vi "SnapCounter_DetectEvent.vi"(3 "status":bool, 4 "error in (no error)":errorcluster, 5 "Task ID":u32) -> (0 "snap counter data":cluster{"event source":i32, "event data":u8[]}, 1 "error out":errorcluster, 2 "Task ID out":u32)   [LabVIEW 2015]
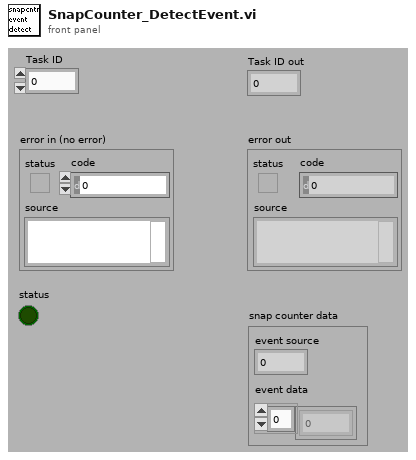
[diagram p1: front panel]
types:
  T1 = cluster{"snap event source":i32, "snap data":i32[]}
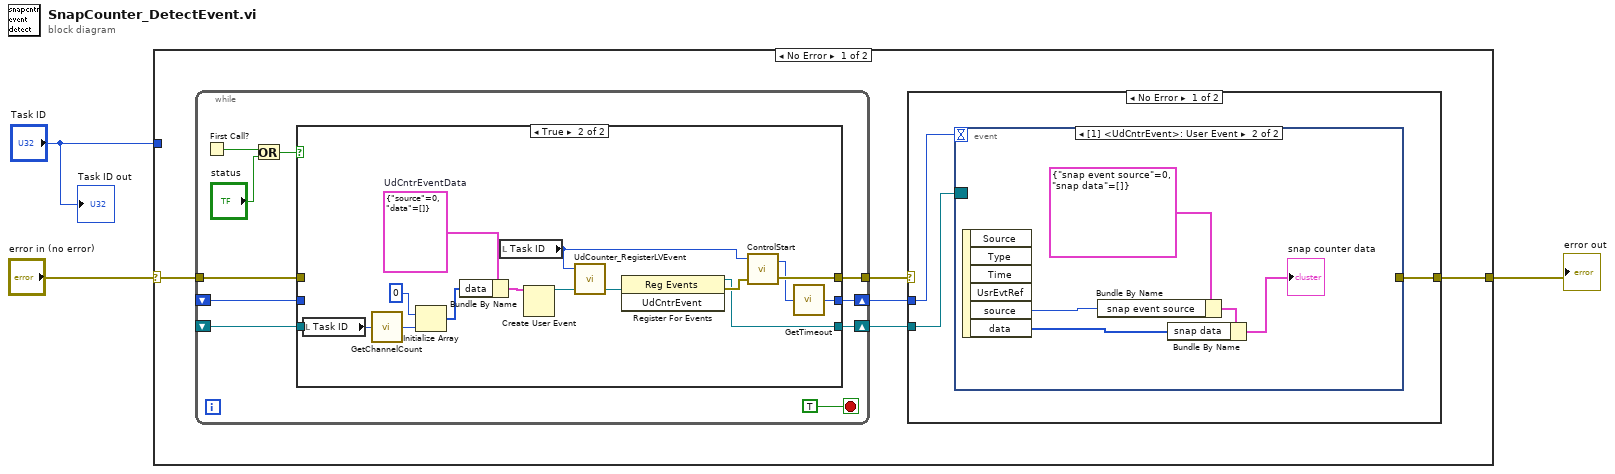
[diagram p0: block diagram]
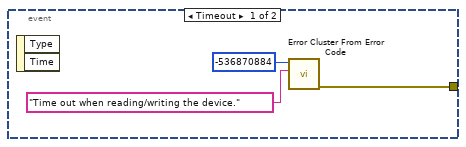
[diagram p2: hidden frame]
diagram:
  n1 = case shown="No Error" "error in (no error)" {
    selector: "error in (no error)" -> [w8 w48]
    tunnel: [w6 w48] -> w2
    tunnel: "Task ID" -> [_ _]
    frame No Error {
      n2 = while {
        tunnel: w8 -> [w26]
        tunnel: [w25] -> w7
        shift-right: [w23] -> w4
        shift-left: _ -> [w24]
        shift-right: [w21] -> w5
        shift-left: _ -> [w22]
        stop <- TRUE stop-if-true
        n3 = First Call?() -> (First Call?: T/F=w29:bool)
        n4 = Or(x=w29, y="status") -> (x .or. y?=w27:bool)
        n5 = case shown="True" w27 {
          tunnel: w26 -> [w33 _]
          tunnel: [w33 w40] -> w25
          tunnel: w24 -> [w32 _]
          tunnel: [w32 w39] -> w23
          tunnel: [w31 w38] -> w21
          tunnel: w22 -> [w31 _]
          frame False {
          }
          frame True {
            w44 = cluster{"source":i64, "data":i32[]} {"source"=0, "data"=[]}  # UdCntrEventData
            n6 = local read "Task ID"() -> (w47:u32)
            n7 = call "GetChannelCount.vi"("Task ID"=w47) -> ("return type"=w46:i32)
            n8 = Initialize Array(0 ("element"), w46) -> (w43:i32[])
            n9 = Bundle By Name(cluster=w44, "data"=w43) -> (w42:cluster{"source":i64, "data":i32[]})
            n10 = local read "Task ID"() -> (w36:u32)
            n11 = Create User Event(user event datatype=w42) -> (user event=w35:refnum<user-event>)  [unwired: 1 in, 1 out]
            n12 = call "UdCounter_RegisterLVEvent.vi"("UdCntrEvent"=w35, "Task ID"=w36) -> ("UdCntrEvent"=w34:refnum<user-event>)  [unwired: 1 in, 2 out]
            n13 = register-events(w34) -> (reference out=w39:refnum<event-registration>, error out=w41:errorcluster)  [unwired: 2 in]
            n14 = call "ControlStart.vi"("error in (no error)"=w41, "Task ID"=w36) -> ("error out"=w40:errorcluster, "Task ID"=w37:u32)  [unwired: 1 out]
            n15 = call "GetTimeout.vi"("Task ID"=w37) -> ("return type"=w38:i32)
          }
        }
      }
      n16 = case shown="No Error" w7 {
        selector: w7 -> [_ w20]
        tunnel: [w9 w20] -> w6
        tunnel: w5 -> [w11 _]
        tunnel: w4 -> [w10 _]
        frame No Error {
          n17 = event shown="[1] <UdCntrEvent>: User Event" {
            selector: w10 -> [_ _]
            dyn-events: _ -> [_ _]
            timeout: w11 -> [_ _]
            tunnel: [w13 _] -> w9
            event Timeout {
              n18 = event-data() -> ()  [unwired: 3 out]
              n19 = call <vilib>:"Error Cluster From Error Code.vi"("error message (\"\")"="Time out when reading/writing the device." ("error message (\"\")"), "error code (0)"=-536870884) -> ("error out"=w13:errorcluster)  [unwired: 2 in, 5 out]
            }
            event User Event {
              n20 = event-data() -> ("source"=w18:i64, "data"=w16:i32[])  [unwired: 5 out]
              n21 = Bundle By Name(cluster=T1 {"snap event source"=0, "snap data"=[]}, "snap event source"=w18) -> (w17:T1)
              n22 = Bundle By Name(cluster=w17, "snap data"=w16) -> (→"snap counter data":T1)
            }
          }
        }
        frame Error {
        }
      }
    }
    frame Error {
    }
  }
  "error out" <- w2
  "Task ID out" <- "Task ID"
